vi "Set Oscillators.vi"(2 "Error In":errorcluster) -> (0 "Error Out":errorcluster, 1 "Oscillators":string[](array[string]))   [LabVIEW 2018]
uses:
  Type Defs/Global Action.ctl
  Type Defs/RT Command.ctl
panel:
  # "Set Oscillators ro Default"
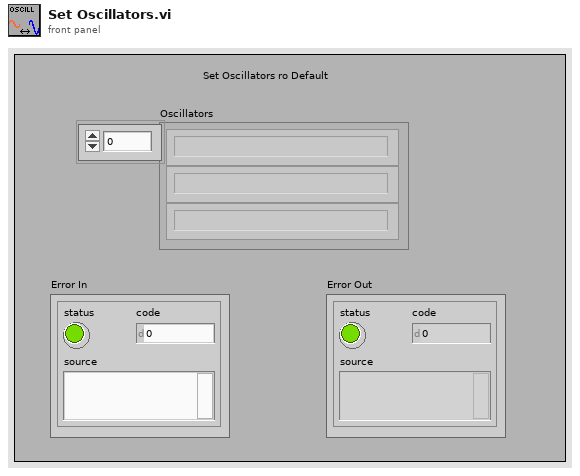
[diagram p1: front panel]
types:
  T1 = typedef "Global Action.ctl" = enum16{"Write", "Read"}
  T2 = typedef "Global Configrations.ctl" = cluster{"Model Name":enum16{"QSight 110", "QSight 120", "QSight 210", "QSight 220", "QSight 410", "QSight 420", "IONICS 3Q 110", "IONICS 3Q 120", "IONICS 3Q 210", "IONICS 3Q 220", "IONICS 3Q 310", "IONICS 3Q 320", "Simulation (Single Source)", "Simulation (Dual Source)"}, "RunType":u16, "Acquisition State":enum16{"Ready", "Busy", "Waiting"}, "InstrState":enum16{"Initializing", "Mass Spectrometer is Off", "Starting Up", "Turning Power Off", "Going to Standby", "Roughing Pump Ready", "Turning Turbo Off", "Turbo Startup", "Turbopump Ready", "Checking Vacuum", "Going to Ready", "Ready", "Running", "Source Standby", "Lost Communication", "Shutting Down", "Fault", "24V Standby", "Go to 24V Standby", "Turbopump Ready-Waiting"}, "Run Mode":enum16{"MRM (Q1/Q2)", "Q1 Scan", "Q1 SRM", "Q2 Scan", "Q2 SRM", "Product Scan", "Precursor Scan", "Neutral Loss", "Neutral Gain"}, "Configration":T3, "TCP ID":refnum<k5>, "DT":bool, "Dead Time (nS)":i32, "Single Source":bool, "ADC Tables":T5[], "FW Udate":bool, "Simulator":bool}
  T3 = typedef "Configration.ctl" = cluster{"Table":T4[], "Instrument":string[]}
  T4 = typedef "Function Lib.lvlib/_RT Configuration 2.ctl" = cluster{"Name":string, "Ch#":u8, "Min":dbl, "Max":dbl, "Def+":dbl, "Def-":dbl, "Offset":dbl, "Slope":dbl, "Type":u8, "Description":string, "SettleT":dbl}
  T5 = typedef "ADC Table.ctl" = cluster{"Name":string, "Ch#":u8, "Min":dbl, "Max":dbl, "Def+":dbl, "Def-":dbl, "Offset":dbl, "Slope":dbl, "Type":u8, "Description":string, "SettleT":dbl}
  T6 = typedef "RT Command.ctl" = enum16{"xml Start Run", "xml Start Actual Run", "xml Stop Run", "xml Runtime Update", "xml Get Status", "xml Get Table", "xml Set Table", "xml Get Configuration", "xml System Status", "xml Set LC Input Logic", "xml Get Data", "xml Get Info", "Start", "StartActualRun", "Stop", "Runtime Update", "Get Data", "Get Info", "Get Status", "Get Param", "Get Config", "Get Table", "Read ADC", "Set Oscillator", "Update Config", "Update Table", "Set All Pol", "Set Pol and DC", "Set Max Mass", "Toggle RP", "Toggle EL", "Set PIC", "Initialize Turbo", "Send Turbo Comm", "Close Turbo", "P1", "P2", "P3", "Send Serial", "Set LC Out", "Get LC In", "Read VAC", "Test Table", "Toggle Power", "Get Startup", "Set Startup", "Get ADC Table", "Set ADC Table", "Get Brief Status", "Get Detail Status", "Auxiliary Update", "Set CC Logics", "Set CC Input Logics", "Ignore Error", "invalid"}
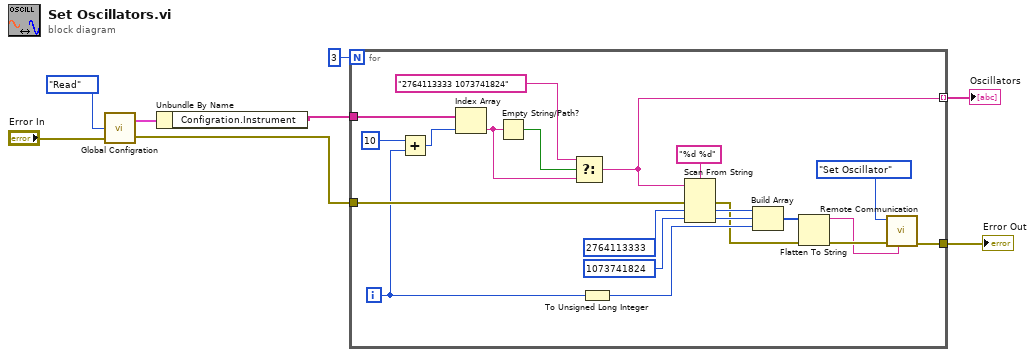
[diagram p0: block diagram]
diagram:
  n1 = call "Global Configration.vi"("Error In"="Error In", "Action"=Global_Action."Read") -> ("Error Out"=w6:errorcluster, "Parameters Out"=w8:T2)  [unwired: 1 in]
  n2 = Unbundle By Name(w8) -> ("Configration.Instrument"=w7:string[])
  n3 = for {
    N: 3 -> [_]
    tunnel: w7 -> [w18]
    tunnel: w6 -> [w17]
    tunnel: [w11] -> w1
    tunnel: [w10] -> w4 mode=indexing
    i -> [w15]
    n4 = Add(x=10 ("y"), y=w15) -> (x+y=w29:i32)
    n5 = Index Array(array=w18, index=w29) -> (element=w27:string)
    n6 = Empty String/Path?(string/path=w27) -> (empty?=w28:bool)
    n7 = Select(t="2764113333 1073741824", s=w28, f=w27) -> (s? t:f=w10:string)
    n8 = To Unsigned Long Integer(number=w15) -> (unsigned 32bit integer=w20:u32)
    n9 = Scan From String(format string="%d %d", input string=w10, error in=w17, default 1=u32 2764113333 ("default value 1"), default 2=u32 1073741824 ("default value 1")) -> (error out=w14:errorcluster, output 1=w22:u32, output 2=w21:u32)  [unwired: 1 in, 2 out]
    n10 = Build Array(w22, w21, w20) -> (w19:u32[])
    n11 = Flatten To String(anything=w19, error in (no error)=w14) -> (data string=w9:string, error out=w13:errorcluster)  [unwired: 3 out]
    n12 = call "Remote Communication.vi"("String"=w9, "Error In"=w13, "Command"=RT_Command."Set Oscillator") -> ("Error Out"=w11:errorcluster)  [unwired: 3 in, 3 out]
  }
  "Oscillators" <- w4
  "Error Out" <- w1
